vi "Power Spectrum.vi"   [LabVIEW 2020, in "NI_AALPro.lvlib"]
doc: "Computes the <B>Power Spectrum</B>, Sxx, of the input sequence <B>X</B>. Wire data to the <B>X</B> input to determine the polymorphic instance to use or manually select the instance."
uses:
  NI_AALPro.lvlib
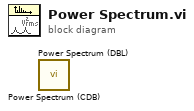
[diagram p0: block diagram]
diagram:
  n1 = call "Power Spectrum (CDB).vi"() -> ()  [unwired: 1 in, 2 out]
  n2 = call "Power Spectrum (DBL).vi"() -> ()  [unwired: 1 in, 2 out]
